vi "SVs.vi"(5 "Data in":dbl[](array[numeric])) -> (3 "G2":dbl[](array[numeric]), 4 "Singular Values":dbl[](graph), 6 "Matrix U":T1, 8 "Matrix S":T1, 10 "Matrix V":T1, 13 "GapCutOff":i16, 14 "Hs":dbl[][](array[numeric]), 15 "SV Gap Ratio":dbl[](array[numeric]))   [LabVIEW 2022 SP3]
uses:
  <vilib>/Analysis/Matrix/Datatypes/RealMatrix.ctl
  <vilib>/Analysis/7linalg.llb/Real SVD Decomposition.vi
  <vilib>/Analysis/NI_AALPro.lvlib
  <vilib>/Analysis/Matrix/NI_Matrix.lvlib
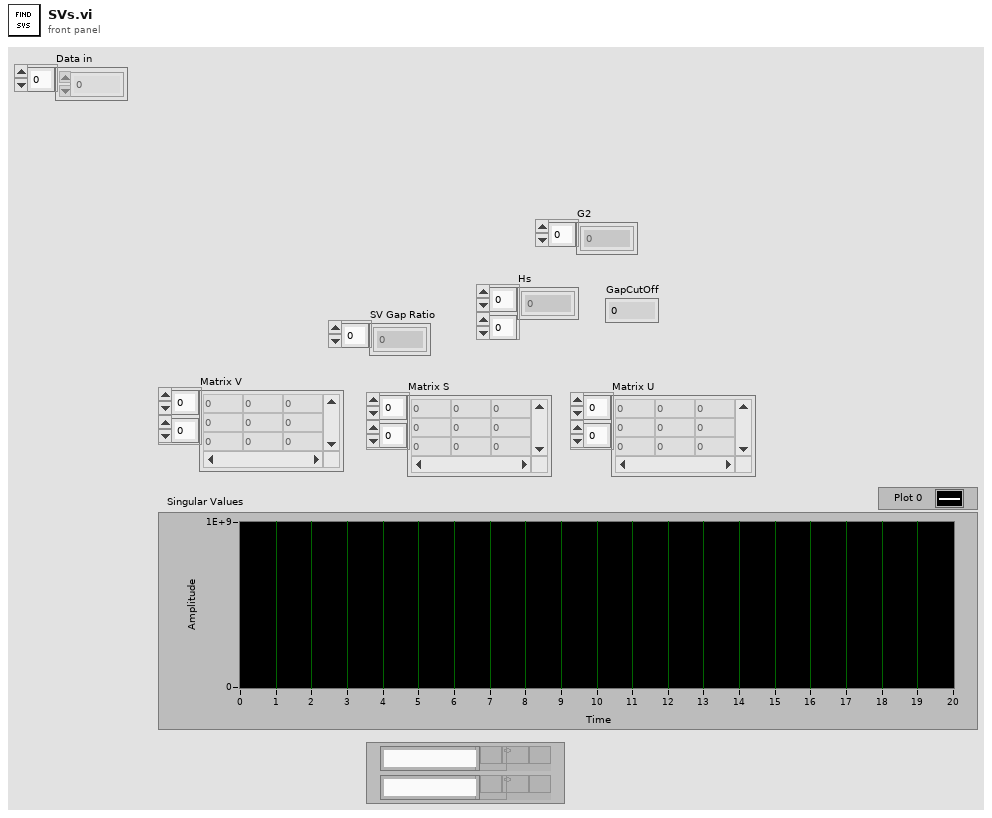
[diagram p1: front panel]
types:
  T1 = typedef "NI_Matrix.lvlib/RealMatrix.ctl" = dbl[][]
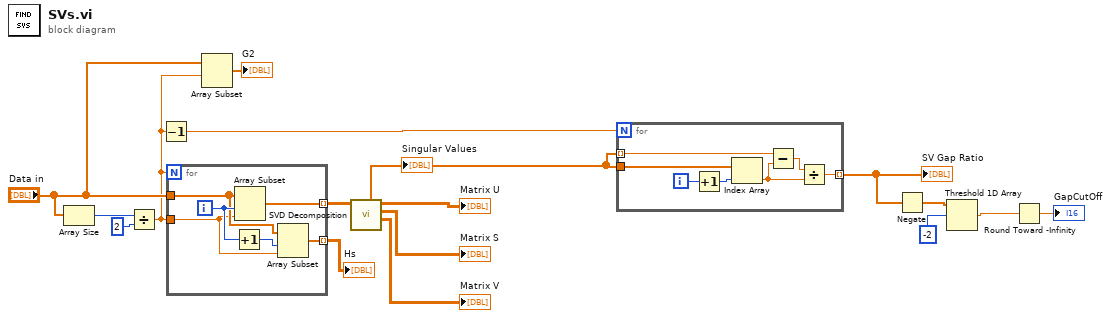
[diagram p0: block diagram]
diagram:
  n1 = Array Size(array="Data in") -> (size(s)=w17:i32)
  n2 = Divide(x=w17, y=2) -> (x/y=w7:dbl)
  n3 = Decrement(x=w7) -> (x-1=w10:dbl)
  n4 = for {
    N: w7 -> [_]
    tunnel: w7 -> [w19]
    tunnel: [w23] -> w16 mode=indexing
    tunnel: "Data in" -> [w20]
    tunnel: [w18] -> w14 mode=indexing
    i -> [w22]
    n5 = Increment(x=w22) -> (x+1=w21:i32)
    n6 = Array Subset(array=w20, index=w22, length=w19) -> (w23:dbl[])
    n7 = Array Subset(array=w20, index=w21, length=w19) -> (w18:dbl[])
  }
  "Hs" <- w14
  n8 = Array Subset(array="Data in", index=w7) -> (→"G2":dbl[])  [unwired: 1 in]
  n9 = call-poly <vilib>:"SVD Decomposition.vi"("A"=w16) -> ("Matrix V"=→"Matrix V":T1, "Matrix S"=→"Matrix S":T1, "Matrix U"=→"Matrix U":T1, "Vector S"=w9:dbl[])  [unwired: 6 in, 1 out]
  "Singular Values" <- w9
  n10 = for {
    N: w10 -> [_]
    tunnel: w9 -> [w29]
    tunnel: w9 -> [w25] mode=indexing
    tunnel: [w26] -> w5 mode=indexing
    i -> [w30]
    n11 = Increment(x=w30) -> (x+1=w27:i32)
    n12 = Index Array(array=w29, index=w27) -> (element=w24:dbl)
    n13 = Subtract(x=w25, y=w24) -> (x-y=w28:dbl)
    n14 = Divide(x=w28, y=w24) -> (x/y=w26:dbl)
  }
  "SV Gap Ratio" <- w5
  n15 = Negate(x=w5) -> (-x=w4:dbl[])
  n16 = Threshold 1D Array(2:-2, 3:w4) -> (0:w2:dbl)  [unwired: 1 in]
  n17 = Round Toward -Infinity(1:w2) -> (0:→"GapCutOff":dbl)
